vi "Get MCP Voltage.vi"(11 "iVoltage":i32) -> (2 "function return":u32, 3 "iVoltage out":i32)   [LabVIEW 2018, in "AndorSDK.lvlib"]
doc: "EXPNETTYPE unsigned int WINAPI GetMCPVoltage(int * iVoltage);"
uses:
  AndorSDK.lvlib
  ATMCD32D.dll
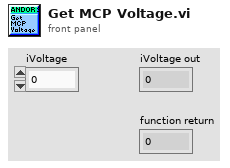
[diagram p1: front panel]
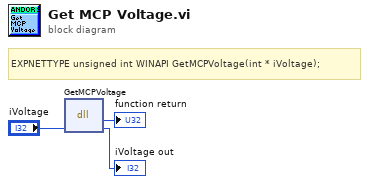
[diagram p0: block diagram]
diagram:
  # "EXPNETTYPE unsigned int WINAPI GetMCPVoltage(int * iVoltage);"
  n1 = dll-call lib="PTH2babs E\nPersönliches02 - Arbeit03-HiwijobsLabviewCodelibANDOR\tAndor SDK\nATMCD32D.*" fn="GetMCPVoltage"("iVoltage"="iVoltage") -> (→"function return":u32, "iVoltage"=→"iVoltage out":i32)  [unwired: 3 in, 2 out]
